vi "Convert U8 Array to Bool Array.vi"(7 "U8 array in":u8[](array[numeric]) format="%.0b") -> (8 "Boolean array out":bool[](array[boolean]))   [LabVIEW 2020]
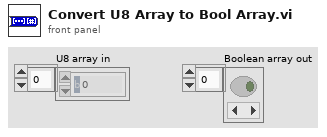
[diagram p1: front panel]
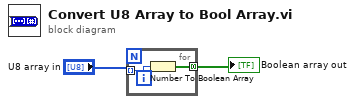
[diagram p0: block diagram]
diagram:
  n1 = for {
    tunnel: "U8 array in" -> [w4] mode=indexing
    tunnel: [w3] -> w1 mode=concatenating
    n2 = Number To Boolean Array(number=w4) -> (Boolean array=w3:bool[])
  }
  "Boolean array out" <- w1
